vi "settingsManagerBackEnd.vi"(8 "error in (no error)":errorcluster, 11 "SettingsManager in":refnum<class "SettingsManager.lvclass">) -> (0 "error out":errorcluster, 3 "SettingsManager out":refnum<class "SettingsManager.lvclass">)   [LabVIEW 2011, in "Tools.lvlib" / "Settings.lvlib" / "SettingsManager.lvclass"]
uses:
  SettingsManager.lvclass
  SettingsEventManager/SettingsEventsManager.lvclass
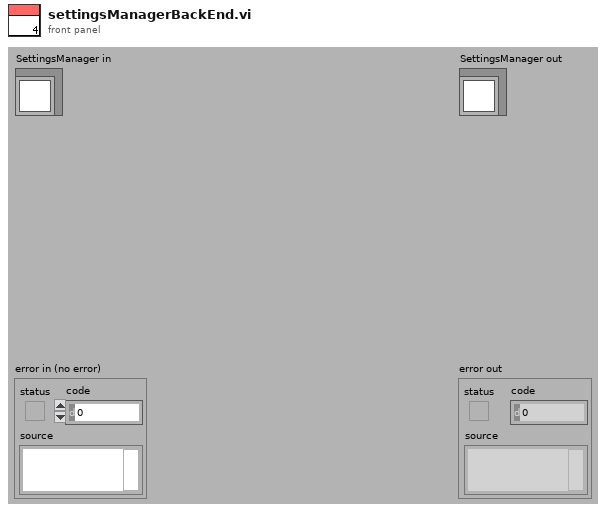
[diagram p1: front panel]
types:
  T1 = enum16{"Number", "String", "NumberArray", "StringArray"}
  T2 = enum16{"Number", "String", "NumberArray", "StringArray", "xmlNode"}
  T3 = cluster{"settingsFrontEndEvents":cluster{"loadSettingsFromPath":refnum<user-event>, "lookUpElementEvent":refnum<user-event>, "saveSettings":refnum<user-event>, "loadSettings":refnum<user-event>, "close":refnum<user-event>, "replaceElement":refnum<user-event>, "findParentNodes":refnum<user-event>, "createNode":refnum<user-event>}, "settingBackEndEvents":cluster{"defaultSettingsPathRequest":refnum<user-event>, "searchResultEvent":refnum<user-event>, "settingsSaved":refnum<user-event>, "settingsLoaded":refnum<user-event>, "foundParentNode":refnum<user-event>}}
  T4 = cluster{"defaultSettingsPathRequest":refnum<user-event>, "searchResultEvent":refnum<user-event>, "settingsSaved":refnum<user-event>, "settingsLoaded":refnum<user-event>, "foundParentNode":refnum<user-event>}
  T5 = cluster{"loadSettingsFromPath":refnum<user-event>, "lookUpElementEvent":refnum<user-event>, "saveSettings":refnum<user-event>, "loadSettings":refnum<user-event>, "close":refnum<user-event>, "replaceElement":refnum<user-event>, "findParentNodes":refnum<user-event>, "createNode":refnum<user-event>}
  T6 = cluster{"lookUpElement":string, "typeEnum":enum16{"Number", "String", "NumberArray", "StringArray"}, "Variant":variant, "lookUpInElement":string}
  T7 = cluster{"lookUpElement":string, "typeEnum":enum16{"Number", "String", "NumberArray", "StringArray", "xmlNode"}, "Variant":variant, "lookUpInElement":string}
  T8 = cluster{"parentNodePaths":string[], "searchElement":string, "type":enum16{"element", "attribute", "value"}, "searchIn":string}
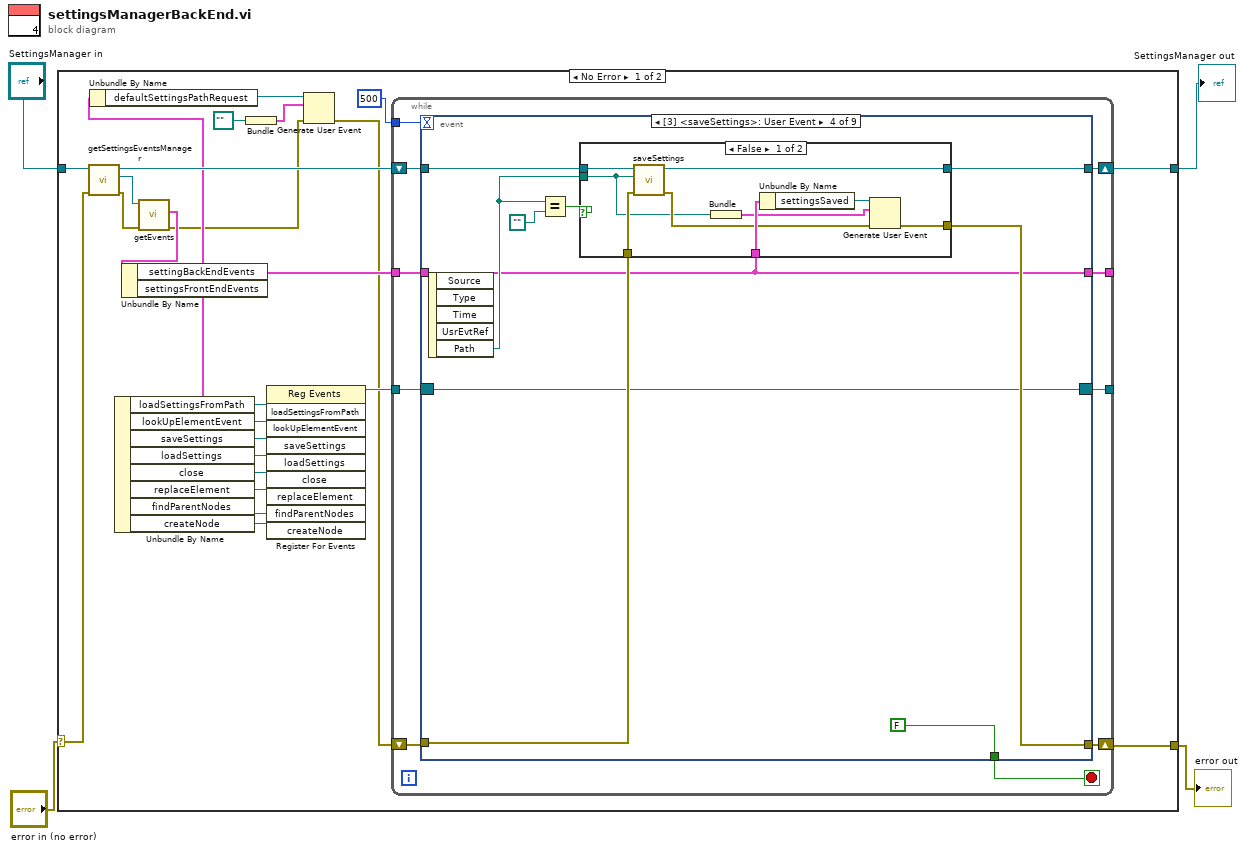
[diagram p0: block diagram]
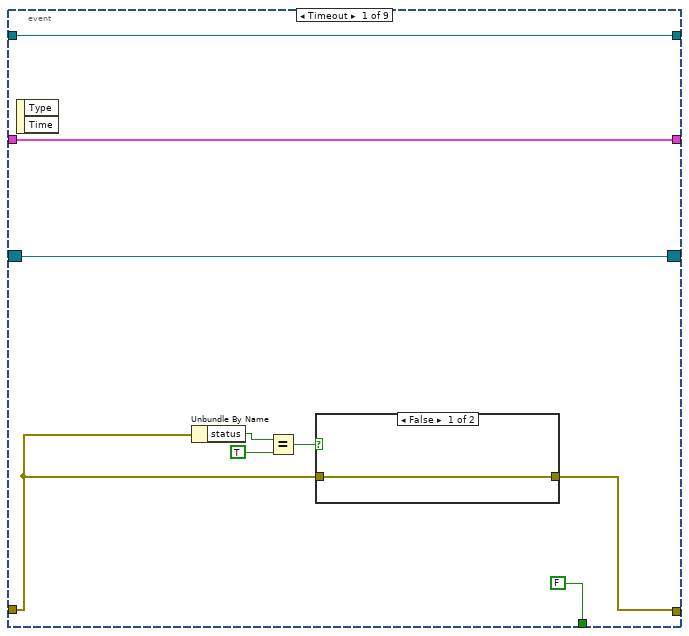
[diagram p2: hidden frame]
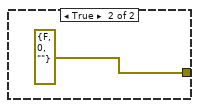
[diagram p3: hidden frame]
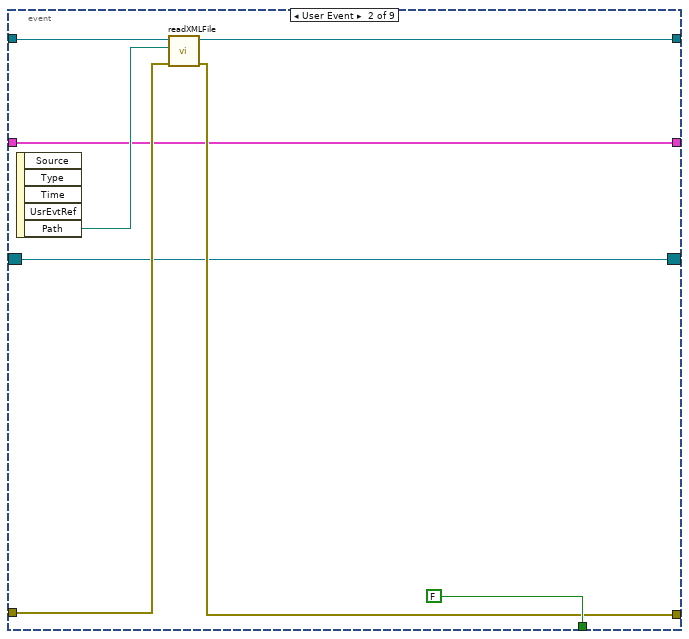
[diagram p4: hidden frame]
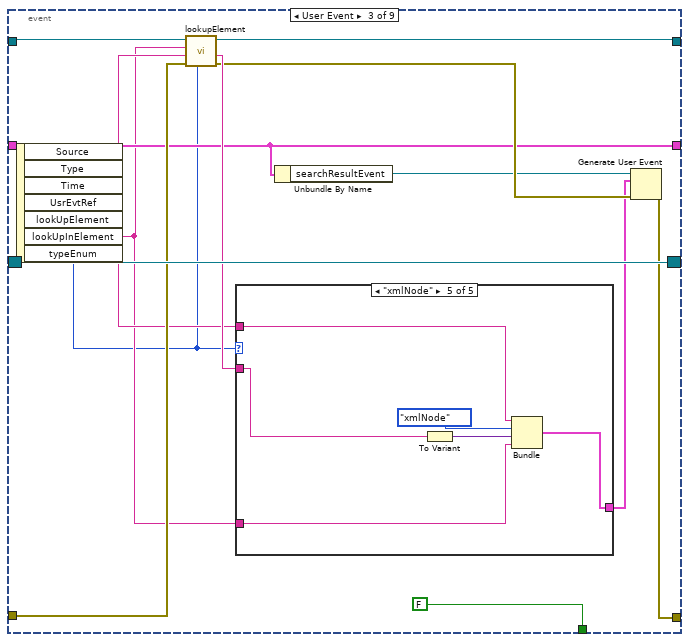
[diagram p5: hidden frame]
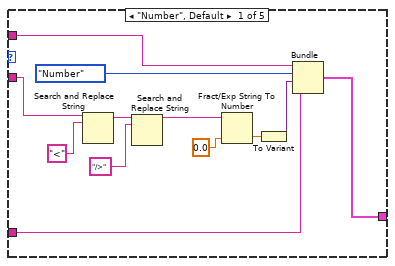
[diagram p6: hidden frame]
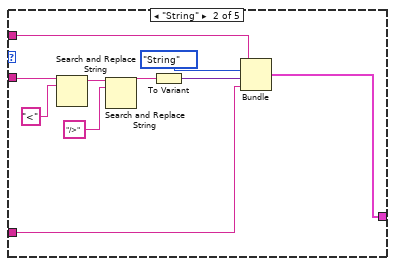
[diagram p7: hidden frame]
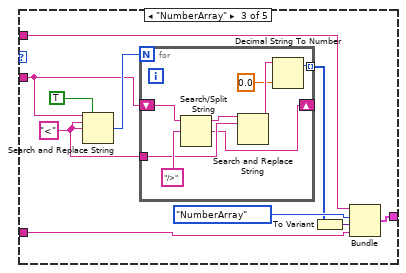
[diagram p8: hidden frame]
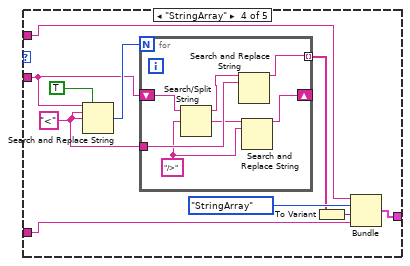
[diagram p9: hidden frame]
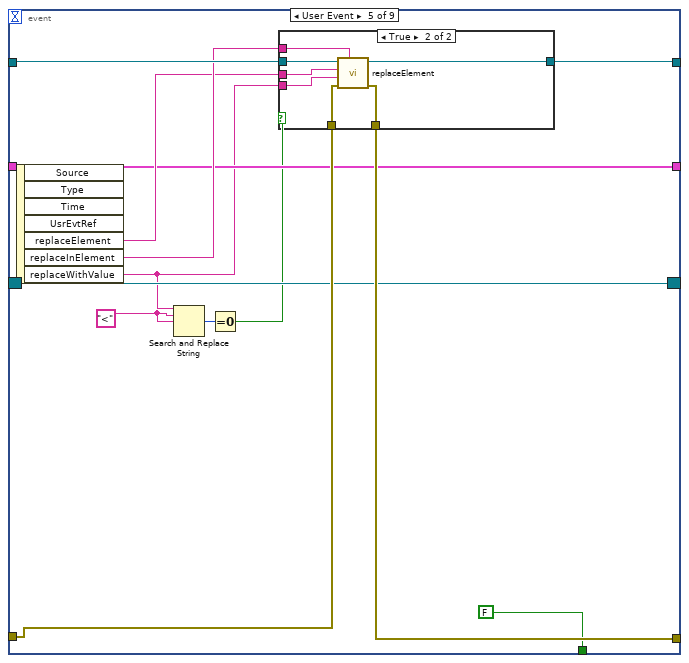
[diagram p11: hidden frame]
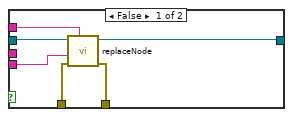
[diagram p12: hidden frame]
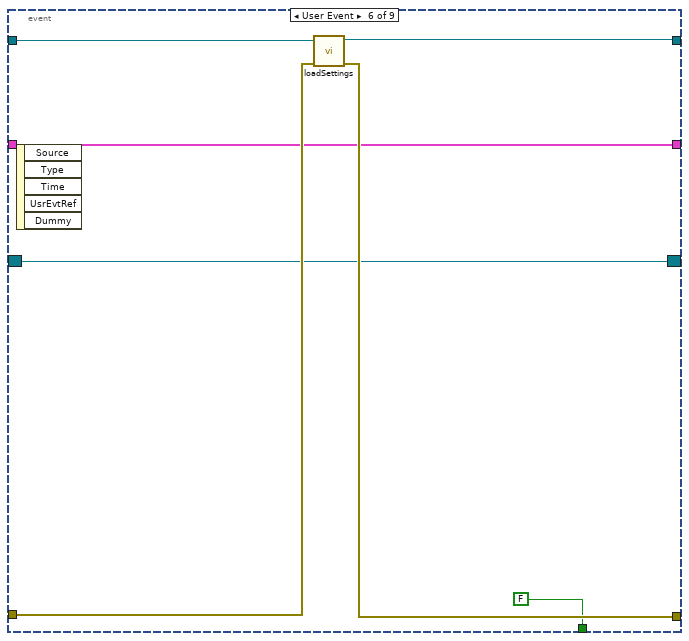
[diagram p13: hidden frame]
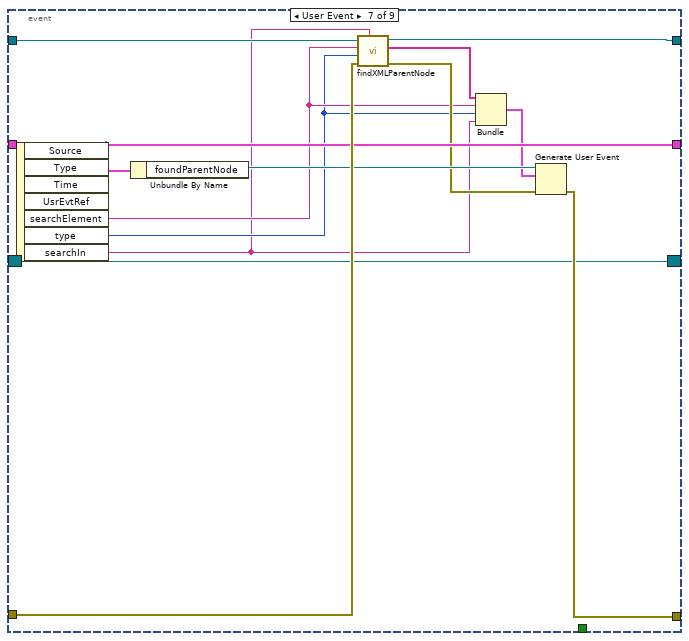
[diagram p14: hidden frame]
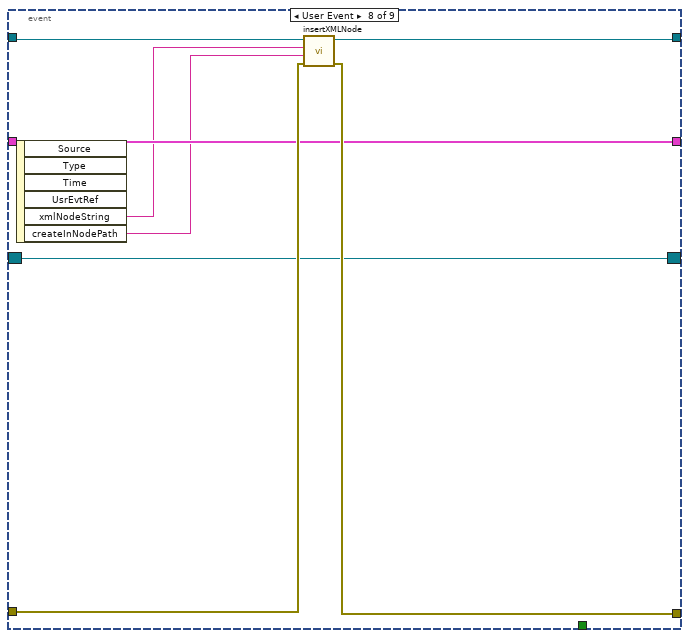
[diagram p15: hidden frame]
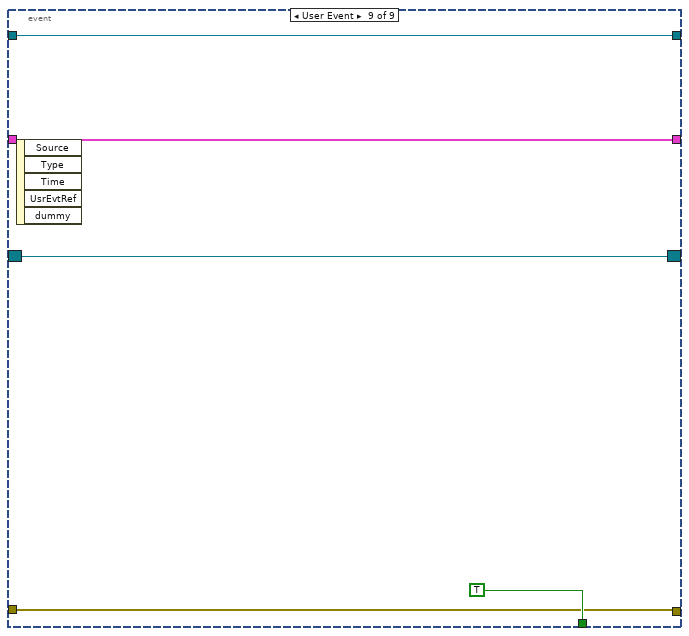
[diagram p16: hidden frame]
diagram:
  n1 = case shown="No Error" "error in (no error)" {
    selector: "error in (no error)" -> [w25 w217]
    tunnel: [w24 w217] -> w3
    tunnel: [w26 w216] -> w1
    tunnel: "SettingsManager in" -> [w29 w216]
    frame No Error {
      n2 = call-dynamic "getSettingsEventsManager.vi"("error in (no error)"=w25, "SettingsManager.lvclass in"=w29) -> ("error out"=w22:errorcluster, "Tools.lvlib:Settings.lvlib:SettingsEventsManager.lvclass"=w23:refnum<class "SettingsEventsManager.lvclass">, "SettingsManager.lvclass out"=w27:refnum<class "SettingsManager.lvclass">)  [unwired: 7 in]
      n3 = call-dynamic "getEvents.vi"("error in (no error)"=w22, "SettingsEventsManager in"=w23) -> ("error out"=w7:errorcluster, "settingsEvents"=w21:T3)  [unwired: 7 in, 1 out]
      n4 = Unbundle By Name(w21) -> ("settingBackEndEvents"=w11:T4, "settingsFrontEndEvents"=w20:T5)
      n5 = Unbundle By Name(w11) -> ("defaultSettingsPathRequest"=w10:refnum<user-event>)
      n6 = Unbundle By Name(w20) -> ("loadSettingsFromPath"=w19:refnum<user-event>, "lookUpElementEvent"=w18:refnum<user-event>, "saveSettings"=w17:refnum<user-event>, "loadSettings"=w16:refnum<user-event>, "close"=w15:refnum<user-event>, "replaceElement"=w14:refnum<user-event>, "findParentNodes"=w13:refnum<user-event>, "createNode"=w12:refnum<user-event>)
      n7 = Bundle(path "") -> (w8:cluster{path})  [unwired: 1 in]
      n8 = register-events(w19, w18, w17, w16, w15, w14, w13, w12) -> (reference out=w28:refnum<event-registration>)  [unwired: 2 in, 1 out]
      n9 = Generate User Event(user event=w10, event data cluster=w8, error in=w7) -> (error out=w6:errorcluster)  [unwired: 1 out]
      n10 = while {
        tunnel: w11 -> [w39]
        tunnel: w28 -> [w38]
        tunnel: [w37] -> _
        tunnel: [w36] -> _
        shift-right: [w34] -> w24
        shift-left: w6 -> [w35]
        shift-right: [w31] -> w26
        shift-left: w27 -> [w33]
        tunnel: 500 -> [w30]
        stop <- w32 stop-if-true
        n11 = event shown="[3] <saveSettings>: User Event" {
          selector: w38 -> [w47 w53 w72 w141 w161 w184 w191 w206 w214]
          dyn-events: [w47 w53 w72 w141 w161 w184 w191 w206 w214] -> w36
          timeout: w30 -> [_ _ _ _ _ _ _ _ _]
          tunnel: w39 -> [w48 w52 w64 w136 w162 w185 w198 w205 w211]
          tunnel: [w48 w52 w64 w136 w162 w185 w198 w205 w211] -> w37
          tunnel: w35 -> [w41 w56 w71 w144 w165 w187 w200 w208 w212]
          tunnel: [w40 w55 w65 w143 w166 w186 w192 w207 w212] -> w34
          tunnel: w33 -> [w46 w57 w60 w145 w169 w189 w202 w210 w213]
          tunnel: [w46 w51 w70 w142 w163 w188 w201 w209 w213] -> w31
          tunnel: [FALSE FALSE FALSE FALSE FALSE FALSE _ _ TRUE] -> w32
          event Timeout {
            n12 = event-data() -> ()  [unwired: 1 in, 2 out]
            n13 = Unbundle By Name(w41) -> ("status"=w42:bool)
            n14 = Equal?(x=w42, y=TRUE) -> (x = y?=w43:bool)
            n15 = case shown="False" w43 {
              tunnel: w41 -> [w49 _]
              tunnel: [w49 errorcluster {"status"=FALSE, "code"=0, "source"=""} ("error out")] -> w40
              frame False {
              }
              frame True {
              }
            }
          }
          event User Event {
            n16 = event-data() -> ("Path"=w54:path)  [unwired: 1 in, 4 out]
            n17 = call "readXMLFile.vi"("error in (no error)"=w56, "Path"=w54, "SettingsManager in"=w57) -> ("error out"=w55:errorcluster, "SettingsManager out"=w51:refnum<class "SettingsManager.lvclass">)  [unwired: 7 in]
          }
          event User Event {
            n18 = event-data() -> ("lookUpElement"=w67:string, "lookUpInElement"=w61:string, "typeEnum"=w59:T2)  [unwired: 1 in, 4 out]
            n19 = call "lookupElement.vi"("typeEnum"=w59, "error in (no error)"=w71, "serachElement"=w67, "searchInElement"=w61, "SettingsManager in"=w60) -> ("error out"=w66:errorcluster, "returnedElements"=w68:string, "SettingsManager out"=w70:refnum<class "SettingsManager.lvclass">)  [unwired: 4 in]
            n20 = case shown="\"xmlNode\"" w59 {
              tunnel: w68 -> [w76 w92 w102 w116 w132]
              tunnel: [w80 w86 w97 w115 w130] -> w63
              tunnel: w67 -> [w81 w93 w100 w117 w133]
              tunnel: w61 -> [w73 w85 w95 w113 w131]
              frame "Number", Default {
                n21 = Search and Replace String(input string=w76, search string="<") -> (result string=w78:string)  [unwired: 6 in, 3 out]
                n22 = Search and Replace String(input string=w78, search string="/>") -> (result string=w75:string)  [unwired: 6 in, 3 out]
                n23 = Fract/Exp String To Number(string=w75, default (0 dbl)=0.0) -> (number=w82:dbl)  [unwired: 2 in, 1 out]
                n24 = To Variant(anything=w82) -> (Variant=w74:variant)
                n25 = Bundle("lookUpElement"=w81, "typeEnum"=T1."Number", "Variant"=w74, "lookUpInElement"=w73) -> (w80:T6)  [unwired: 1 in]
              }
              frame "String" {
                n26 = Search and Replace String(input string=w92, search string="<") -> (result string=w90:string)  [unwired: 6 in, 3 out]
                n27 = Search and Replace String(input string=w90, search string="/>") -> (result string=w88:string)  [unwired: 6 in, 3 out]
                n28 = To Variant(anything=w88) -> (Variant=w87:variant)
                n29 = Bundle("lookUpElement"=w93, "typeEnum"=T1."String", "Variant"=w87, "lookUpInElement"=w85) -> (w86:T6)  [unwired: 1 in]
              }
              frame "NumberArray" {
                w101 = "<"
                n30 = Search and Replace String(replace all?=TRUE, input string=w102, search string=w101, replace string=w101) -> (number of replacements=w103:i32)  [unwired: 4 in, 3 out]
                n31 = for {
                  N: w103 -> [_]
                  tunnel: w101 -> [w110]
                  shift-right: [w109] -> _
                  shift-left: w102 -> [w108]
                  tunnel: [w105] -> w98 mode=indexing
                  n32 = Search/Split String(string=w108, search string/char (-)="/>") -> (substring before match=w111:string, match + rest of string=w109:string)  [unwired: 1 in, 1 out]
                  n33 = Search and Replace String(input string=w111, search string=w110) -> (result string=w107:string)  [unwired: 6 in, 3 out]
                  n34 = Decimal String To Number(string=w107, default (0L)=0.0) -> (offset past number=w105:i32)  [unwired: 1 in, 1 out]
                }
                n35 = To Variant(anything=w98) -> (Variant=w96:variant)
                n36 = Bundle("lookUpElement"=w100, "typeEnum"=T1."NumberArray", "Variant"=w96, "lookUpInElement"=w95) -> (w97:T6)  [unwired: 1 in]
              }
              frame "StringArray" {
                w120 = "<"
                n37 = Search and Replace String(replace all?=TRUE, input string=w116, search string=w120, replace string=w120) -> (number of replacements=w121:i32)  [unwired: 4 in, 3 out]
                n38 = for {
                  N: w121 -> [_]
                  tunnel: w120 -> [w128]
                  shift-right: [w123] -> _
                  shift-left: w116 -> [w127]
                  tunnel: [w126] -> w118 mode=indexing
                  w124 = "/>"
                  n39 = Search/Split String(string=w127, search string/char (-)=w124) -> (substring before match=w129:string, match + rest of string=w125:string)  [unwired: 1 in, 1 out]
                  n40 = Search and Replace String(input string=w129, search string=w128) -> (result string=w126:string)  [unwired: 6 in, 3 out]
                  n41 = Search and Replace String(input string=w125, search string=w124) -> (result string=w123:string)  [unwired: 6 in, 3 out]
                }
                n42 = To Variant(anything=w118) -> (Variant=w114:variant)
                n43 = Bundle("lookUpElement"=w117, "typeEnum"=T1."StringArray", "Variant"=w114, "lookUpInElement"=w113) -> (w115:T6)  [unwired: 1 in]
              }
              frame "xmlNode" {
                n44 = To Variant(anything=w132) -> (Variant=w134:variant)
                n45 = Bundle("lookUpElement"=w133, "typeEnum"=T2."xmlNode", "Variant"=w134, "lookUpInElement"=w131) -> (w130:T7)  [unwired: 1 in]
              }
            }
            n46 = Unbundle By Name(w64) -> ("searchResultEvent"=w62:refnum<user-event>)
            n47 = Generate User Event(user event=w62, event data cluster=w63, error in=w66) -> (error out=w65:errorcluster)  [unwired: 1 out]
          }
          event User Event {
            n48 = event-data() -> ("Path"=w139:path)  [unwired: 1 in, 4 out]
            n49 = Equal?(x=w139, y=path "") -> (x = y?=w138:bool)
            n50 = case shown="False" w138 {
              tunnel: w145 -> [w154 w155]
              tunnel: w144 -> [w153 w156]
              tunnel: [w148 w156] -> w143
              tunnel: [w152 w155] -> w142
              tunnel: w139 -> [w147 _]
              tunnel: w136 -> [w150 _]
              frame False {
                n51 = call "saveSettings.vi"("error in (no error)"=w153, "Path"=w147, "SettingsManager in"=w154) -> ("error out"=w149:errorcluster, "SettingsManager out"=w152:refnum<class "SettingsManager.lvclass">)  [unwired: 7 in]
                n52 = Bundle("Path"=w147) -> (w146:cluster{"Path":path})  [unwired: 1 in]
                n53 = Unbundle By Name(w150) -> ("settingsSaved"=w151:refnum<user-event>)
                n54 = Generate User Event(user event=w151, event data cluster=w146, error in=w149) -> (error out=w148:errorcluster)  [unwired: 1 out]
              }
              frame True {
              }
            }
          }
          event User Event {
            w159 = "<"
            n55 = event-data() -> ("replaceElement"=w167:string, "replaceInElement"=w168:string, "replaceWithValue"=w160:string)  [unwired: 1 in, 4 out]
            n56 = Search and Replace String(input string=w160, search string=w159, replace string=w159) -> (number of replacements=w157:i32)  [unwired: 5 in, 3 out]
            n57 = Equal To 0?(x=w157) -> (x = 0?=w158:bool)
            n58 = case shown="True" w158 {
              tunnel: w169 -> [w175 w182]
              tunnel: w168 -> [w173 w181]
              tunnel: w167 -> [_ w180]
              tunnel: [w170 w179] -> w166
              tunnel: w165 -> [w171 w178]
              tunnel: [w174 w177] -> w163
              tunnel: w160 -> [w172 w176]
              frame False {
                n59 = call "replaceNode.vi"("replaceElementIn"=w173, "error in (no error)"=w171, "replaceWithValue"=w172, "SettingsManager in"=w175) -> ("error out"=w170:errorcluster, "SettingsManager out"=w174:refnum<class "SettingsManager.lvclass">)  [unwired: 6 in]
              }
              frame True {
                n60 = call "replaceElement.vi"("replaceElementIn"=w181, "error in (no error)"=w178, "replaceWithValue"=w176, "replacementElementName"=w180, "SettingsManager in"=w182) -> ("error out"=w179:errorcluster, "SettingsManager out"=w177:refnum<class "SettingsManager.lvclass">)  [unwired: 5 in]
              }
            }
          }
          event User Event {
            n61 = event-data() -> ()  [unwired: 1 in, 5 out]
            n62 = call-dynamic "loadSettings.vi"("error in (no error)"=w187, "SettingsManager in"=w189) -> ("error out"=w186:errorcluster, "SettingsManager out"=w188:refnum<class "SettingsManager.lvclass">)  [unwired: 8 in]
          }
          event User Event {
            n63 = event-data() -> ("searchElement"=w195:string, "type"=w194:enum16{"element", "attribute", "value"}, "searchIn"=w190:string)  [unwired: 1 in, 4 out]
            n64 = Unbundle By Name(w198) -> ("foundParentNode"=w199:refnum<user-event>)
            n65 = call "findXMLParentNode.vi"("searchIn"=w190, "error in (no error)"=w200, "type"=w194, "searchElement"=w195, "SettingsManager in"=w202) -> ("error out"=w197:errorcluster, "parentNodePaths"=w196:string[], "SettingsManager out"=w201:refnum<class "SettingsManager.lvclass">)  [unwired: 4 in]
            n66 = Bundle("parentNodePaths"=w196, "searchElement"=w195, "type"=w194, "searchIn"=w190) -> (w193:T8)  [unwired: 1 in]
            n67 = Generate User Event(user event=w199, event data cluster=w193, error in=w197) -> (error out=w192:errorcluster)  [unwired: 1 out]
          }
          event User Event {
            n68 = event-data() -> ("xmlNodeString"=w204:string, "createInNodePath"=w203:string)  [unwired: 1 in, 4 out]
            n69 = call "insertXMLNode.vi"("error in (no error)"=w208, "createInNodePath"=w203, "xmlNodeString"=w204, "SettingsManager in"=w210) -> ("error out"=w207:errorcluster, "SettingsManager out"=w209:refnum<class "SettingsManager.lvclass">)  [unwired: 6 in]
          }
          event User Event {
            n70 = event-data() -> ()  [unwired: 1 in, 5 out]
          }
        }
      }
    }
    frame Error {
    }
  }
  "error out" <- w3
  "SettingsManager out" <- w1
